vi "turning_correction2.vi"(9 "Parâmetros Ini 2":T1={"Gyro Port"=0, "Sensor - Left"=3, "Sensor - Right"=2, "     Color \nSensor Port"=1, "Kp Front"=0.5, "Motor speed"=-15, "Distance to street"=0.0, "Motor speed turns"=16, "Kp Curvas"=0.0} {"Kp Front" format="%.3f"; "Color \nSensor Port" items=["Port 1", "Port 2", "Port 3", "Port 4"]; "Sensor - Right" items=["Port 1", "Port 2", "Port 3", "Port 4"]; "Sensor - Left" items=["Port 1", "Port 2", "Port 3", "Port 4"]; "Gyro Port" items=["Port 1", "Port 2", "Port 3", "Port 4"]}, 11 "NXT/EV3":T3) -> (1 "NXT/EV3 2":T3)   [LabVIEW 2016]
uses:
  <vilib>/NXT/Subs/LVHSConnector.ctl
  <vilib>/NXT/LegoClasses/BrickReference/BrickReference.lvclass
  parametros.ctl
  <vilib>/NXT/Block Support/NXT_InputPort.ctl
  <vilib>/NXT/Subs/ColorSensorColors.ctl
  <vilib>/NXT/Block Support/NXT_OutputPort.ctl
  <vilib>/NXT/Dual Mode Library/Display/drawText.vi
  <vilib>/NXT/Dual Mode Library/Sensors/EV3_Gyro_Angle.vi
  <vilib>/NXT/NXTIO Xnodes/NXTIONodeSubVIs/NXTMoveMotors.vi
  <vilib>/NXT/NXTIO Xnodes/NXTIONodeSubVIs/NXTMotorRunDistance.vi
  <vilib>/NXT/NXTIO Xnodes/AddressXNode/NXTIOAddress.xnode
  <vilib>/NXT/NXTIO Xnodes/NXTIOXNode/NXTIO.xnode
panel:
  out "Degrees":sgl
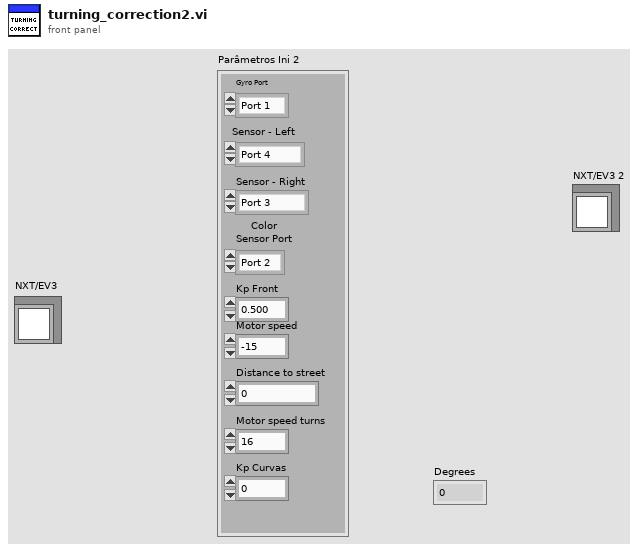
[diagram p1: front panel]
types:
  T1 = typedef "parametros.ctl" = cluster{"Gyro Port":T2, "Sensor - Left":T2, "Sensor - Right":T2, "     Color \nSensor Port":T2, "Kp Front":dbl, "Motor speed":i32, "Distance to street":dbl, "Motor speed turns":i32, "Kp Curvas":dbl}
  T2 = typedef "NXT_InputPort.ctl" = u32
  T3 = typedef "LVHSConnector.ctl" = refnum<class "BrickReference.lvclass">
  T4 = typedef "ColorSensorColors.ctl" = enum16{"No Color", "Black", "Blue", "Green", "Yellow", "Red", "White", "Brown"}
  T5 = typedef "NXT_OutputPort.ctl" = u8
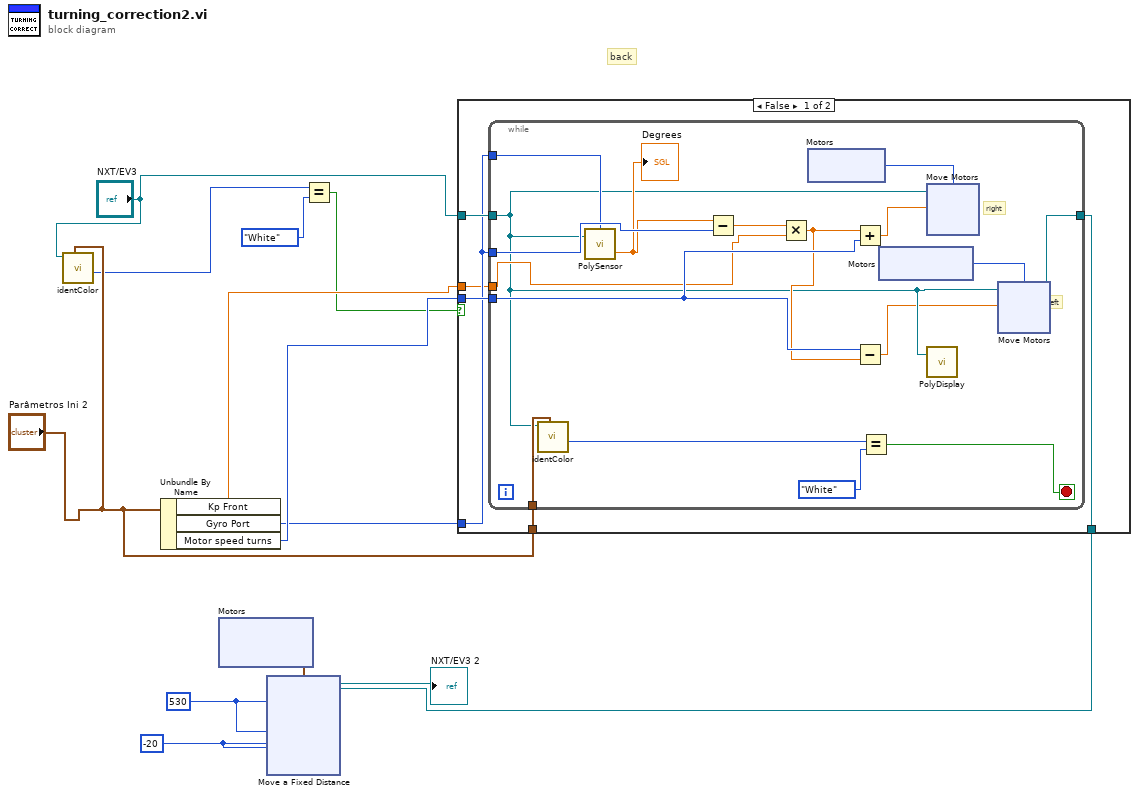
[diagram p0: block diagram]
diagram:
  w11 = i8 -20 ("Speed 1")
  w12 = 530 ("Distance 1")
  # "back"
  n1 = call "identColor.vi"("Parâmetros Ini"="Parâmetros Ini 2", "NXT/EV3"="NXT/EV3") -> ("Collor"=w4:T4)  [unwired: 8 in, 1 out]
  n2 = Unbundle By Name("Parâmetros Ini 2") -> ("Kp Front"=w7:dbl, "Gyro Port"=w8:T2, "Motor speed turns"=w9:i32)
  n3 = xnode "Motors"() -> ("Motor"=w13:cluster{"Port":T5, "Port":T5})
  n4 = Equal?(x=w4, y=ColorSensorColors."White" ("Collor")) -> (x = y?=w1:bool)
  n5 = case shown="False" w1 {
    tunnel: "NXT/EV3" -> [w19 w53]
    tunnel: w9 -> [w18 _]
    tunnel: w8 -> [w17 _]
    tunnel: w7 -> [w16 _]
    tunnel: [w15 w53] -> w6
    tunnel: "Parâmetros Ini 2" -> [w14 _]
    frame False {
      n6 = while {
        tunnel: w17 -> [w36]
        tunnel: w18 -> [w35]
        tunnel: w17 -> [w34]
        tunnel: w16 -> [w33]
        tunnel: w14 -> [w24]
        tunnel: w19 -> [w22]
        tunnel: [w32] -> w15
        stop <- w25 stop-if-true
        # "left"
        # "right"
        n7 = call "identColor.vi"("Parâmetros Ini"=w24, "NXT/EV3"=w22) -> ("Collor"=w23:T4)  [unwired: 8 in, 1 out]
        n8 = call-poly <vilib>:"PolySensor.vi"("NXT/EV3"=w22, "Port (Port 1)"=w34) -> ("Degrees"=w29:sgl)  [unwired: 1 in, 1 out]
        "Degrees" <- w29
        n9 = Subtract(x=w29, y=w36) -> (x-y=w30:sgl)
        n10 = Multiply(x=w30, y=w33) -> (x*y=w31:dbl)
        n11 = xnode "Motors"() -> ("Motor"=w28:T5)
        n12 = Add(x=w31, y=w35) -> (x+y=w21:dbl)
        n13 = Subtract(x=w35, y=w31) -> (x-y=w20:dbl)
        n14 = Equal?(x=w23, y=ColorSensorColors."White" ("Collor")) -> (x = y?=w25:bool)
        n15 = xnode "Motors"() -> ("Motor"=w27:T5)
        n16 = xnode "Move Motors"("Power/Speed 1"=w21, "Motors"=w28, "NXT/EV3"=w22) -> ()  [unwired: 1 out]
        n17 = call-poly <vilib>:"PolyDisplay.vi"("NXT/EV3"=w22) -> ()  [unwired: 3 in, 1 out]
        n18 = xnode "Move Motors"("Power/Speed 1"=w20, "Motors"=w27, "NXT/EV3"=w22) -> ("NXT/EV3"=w32:T3)
      }
    }
    frame True {
    }
  }
  n19 = xnode "Move a Fixed Distance"("Speed 2"=w11, "Speed 1"=w11, "Distance 2"=w12, "Distance 1"=w12, "Motors"=w13, "NXT/EV3"=w6) -> ("NXT/EV3"=→"NXT/EV3 2":T3)
